vi "Utilities-Wait.vi"(7 "milliseconds to wait":dbl, 11 "error in (no error)":errorcluster) -> (15 "error out":errorcluster)   [LabVIEW 2020]
uses:
  89bc9713-8f2c-40bd-a11f-1c800a437687.vi
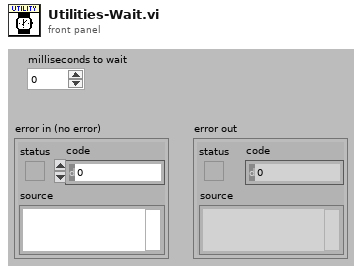
[diagram p1: front panel]
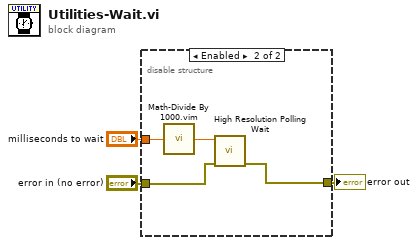
[diagram p0: block diagram]
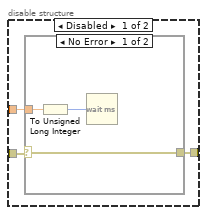
[diagram p2: hidden frame]
diagram:
  n1 = disable-structure shown="Enabled" {
    disable-tunnel: "error in (no error)" -> [w6 w12]
    disable-tunnel: [w5 w11] -> w2
    disable-tunnel: "milliseconds to wait" -> [w4 w14]
    frame Disabled {
      n2 = case shown="No Error" w6 {
        selector: w6 -> [w9 w10]
        tunnel: [w9 w10] -> w5
        tunnel: w4 -> [w8 _]
        frame No Error {
          n3 = To Unsigned Long Integer(number=w8) -> (unsigned 32bit integer=w7:u32)
          n4 = Wait (ms)(milliseconds to wait=w7) -> ()  [unwired: 1 out]
        }
        frame Error {
        }
      }
    }
    frame Enabled {
      n5 = call "Math-Divide By 1000.vim"("X"=w14) -> ("1000X"=w13:dbl)
      n6 = call <vilib>:"High Resolution Polling Wait.vi"("error in (no error)"=w12, "seconds to wait"=w13) -> ("error out"=w11:errorcluster)  [unwired: 9 in]
    }
  }
  "error out" <- w2
